vi "Fuzzy-Output-SubVi-2.0.vi"(0 "Slide in":refnum<vi>, 1 "Slide Refnum 4":refnum<vi>, 2 "Zero Upper Limit":dbl, 3 "Slide Refnum 5":refnum<vi>, 4 "Zero Medium Limit [Fixed]":dbl, 5 "Slide Refnum 6":refnum<vi>, 6 "Slide Refnum 7":refnum<vi>, 8 "Positive Lower Limit [Fixed]":dbl, 9 "Min Err":dbl, 10 "Slide Refnum 3":refnum<vi>, 11 "Negative Lower Limit [Fixed]":dbl, 12 "Positive Upper Limit [Fixed]":dbl, 13 "Negative Upper Limit [Fixed]":dbl, 14 "Slide Refnum in":refnum<vi>, 15 "Zero Lower Limit":dbl, 16 "Max Err":dbl, 18 "Min Intersection":dbl) -> (20 "Array":cluster{dbl[], dbl[]}[](array[cluster]))   [LabVIEW 2016]
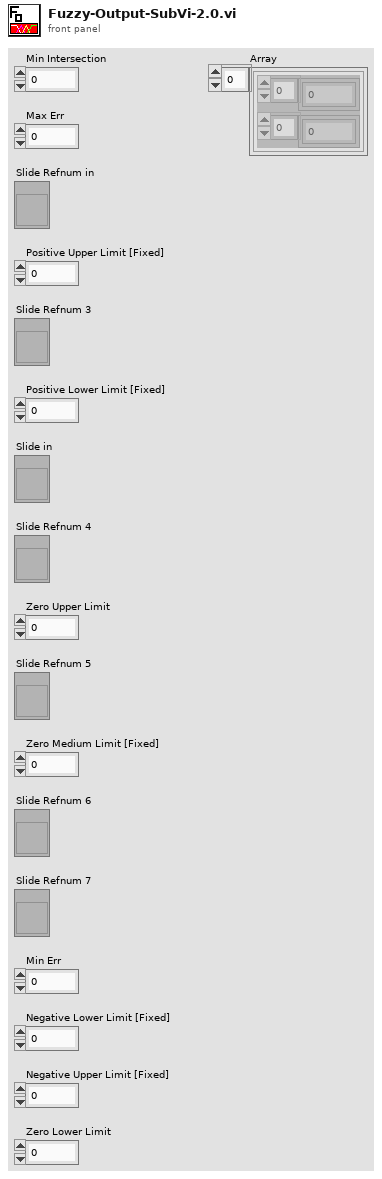
[diagram p1: front panel]
types:
  T1 = enum8{"Enabled", "Disabled", "Disabled and Grayed Out"}
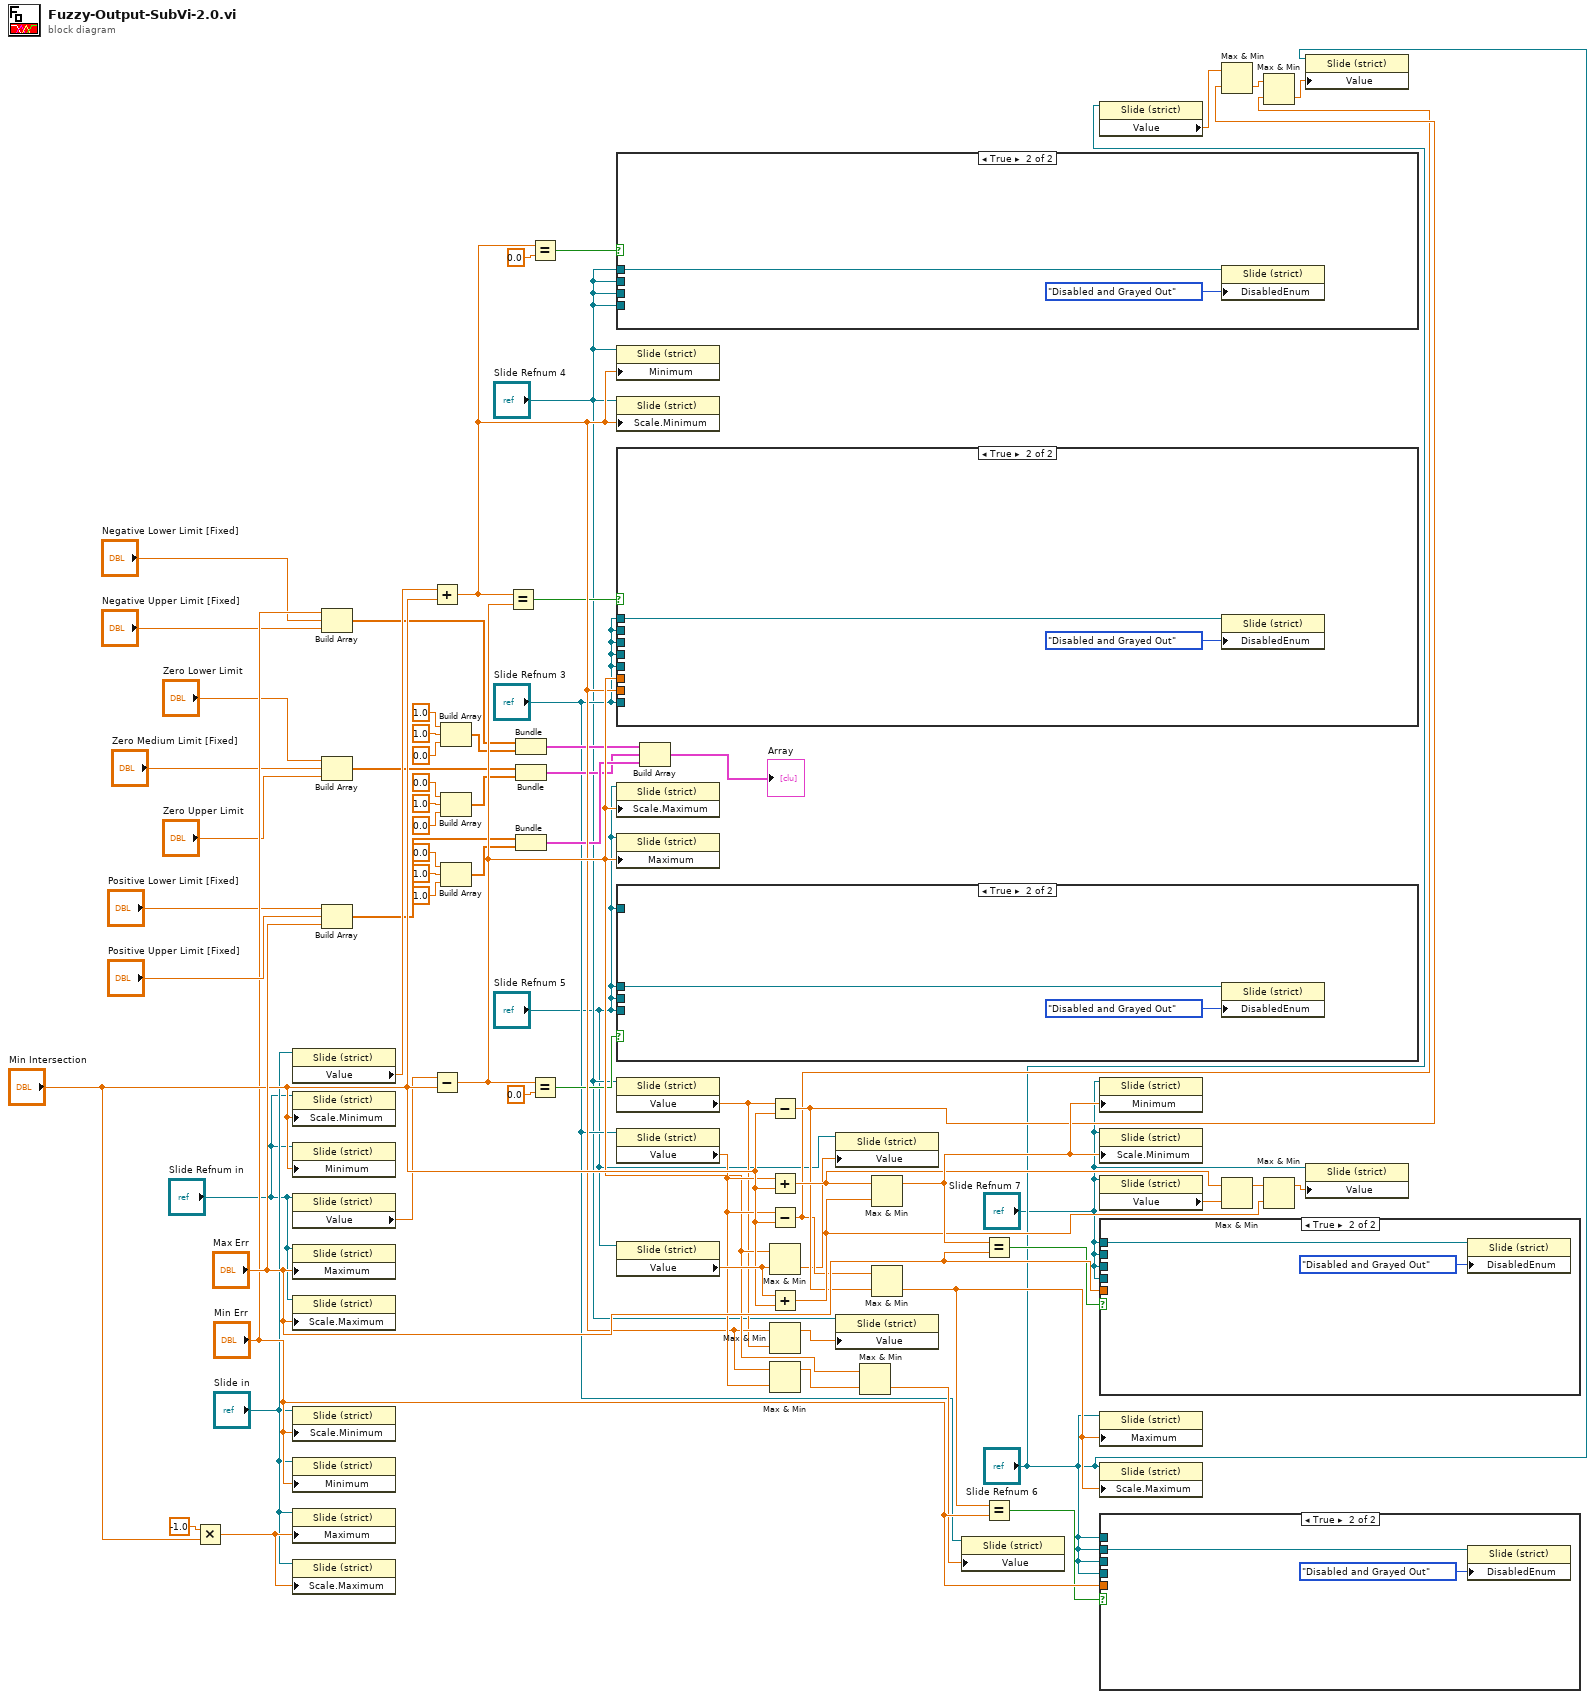
[diagram p0: block diagram]
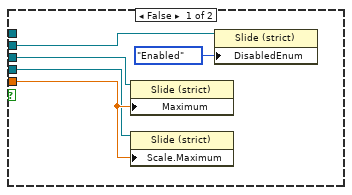
[diagram p2: hidden frame]
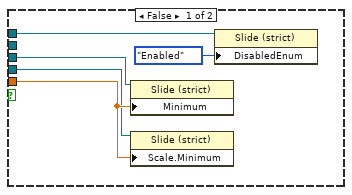
[diagram p3: hidden frame]
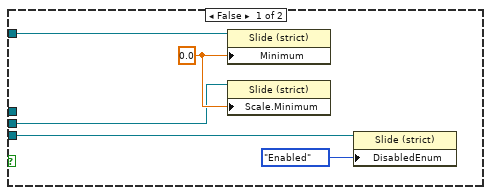
[diagram p4: hidden frame]
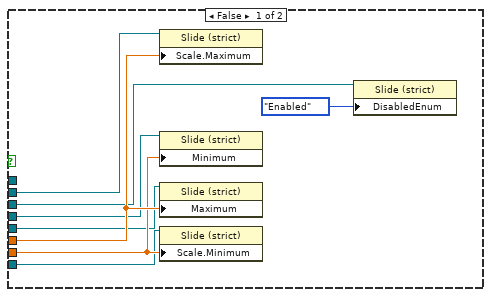
[diagram p5: hidden frame]
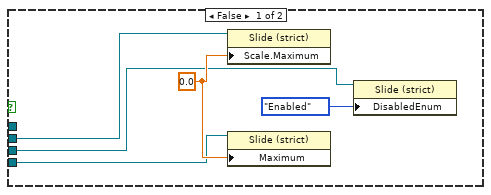
[diagram p6: hidden frame]
diagram:
  n1 = Multiply(x=-1.0, y="Min Intersection") -> (x*y=w54:dbl)
  n2 = property on="Property Node" class="Slide (strict)"(reference="Slide in") -> ("Value"=w32:dbl)  [unwired: 1 in, 2 out]
  n3 = property on="Property Node" class="Slide (strict)"(reference="Slide Refnum in", "Scale.Minimum"="Min Intersection") -> ()  [unwired: 1 in, 2 out]
  n4 = property on="Property Node" class="Slide (strict)"(reference="Slide Refnum in", "Minimum"="Min Intersection") -> ()  [unwired: 1 in, 2 out]
  n5 = property on="Property Node" class="Slide (strict)"(reference="Slide Refnum in") -> ("Value"=w31:dbl)  [unwired: 1 in, 2 out]
  n6 = property on="Property Node" class="Slide (strict)"(reference="Slide Refnum in", "Maximum"="Max Err") -> ()  [unwired: 1 in, 2 out]
  n7 = property on="Property Node" class="Slide (strict)"(reference="Slide Refnum in", "Scale.Maximum"="Max Err") -> ()  [unwired: 1 in, 2 out]
  n8 = property on="Property Node" class="Slide (strict)"(reference="Slide in", "Scale.Minimum"="Min Err") -> ()  [unwired: 1 in, 2 out]
  n9 = property on="Property Node" class="Slide (strict)"(reference="Slide in", "Minimum"="Min Err") -> ()  [unwired: 1 in, 2 out]
  n10 = property on="Property Node" class="Slide (strict)"(reference="Slide in", "Maximum"=w54) -> ()  [unwired: 1 in, 2 out]
  n11 = property on="Property Node" class="Slide (strict)"(reference="Slide in", "Scale.Maximum"=w54) -> ()  [unwired: 1 in, 2 out]
  n12 = Build Array("Min Err", "Negative Lower Limit [Fixed]", "Negative Upper Limit [Fixed]") -> (w10:dbl[])
  n13 = Build Array("Zero Lower Limit", "Zero Medium Limit [Fixed]", "Zero Upper Limit") -> (w18:dbl[])
  n14 = Build Array("Positive Lower Limit [Fixed]", "Positive Upper Limit [Fixed]", "Max Err") -> (w25:dbl[])
  n15 = Add(x=w32, y="Min Intersection") -> (x+y=w52:dbl)
  n16 = Subtract(x=w31, y="Min Intersection") -> (x-y=w55:dbl)
  n17 = Build Array(1.0 ("element"), 1.0 ("element"), 0.0 ("element")) -> (w11:dbl[])
  n18 = Build Array(0.0 ("element"), 1.0 ("element"), 0.0 ("element")) -> (w19:dbl[])
  n19 = Build Array(0.0 ("element"), 1.0 ("element"), 1.0 ("element")) -> (w26:dbl[])
  n20 = Equal?(x=w52, y=w55) -> (x = y?=w36:bool)
  n21 = Bundle(w10, w11) -> (w20:cluster{dbl[], dbl[]})  [unwired: 1 in]
  n22 = Bundle(w18, w19) -> (w21:cluster{dbl[], dbl[]})  [unwired: 1 in]
  n23 = Bundle(w25, w26) -> (w28:cluster{dbl[], dbl[]})  [unwired: 1 in]
  n24 = Equal?(x=w52, y=0.0) -> (x = y?=w35:bool)
  n25 = Equal?(x=w55, y=0.0) -> (x = y?=w39:bool)
  n26 = case shown="True" w35 {
    tunnel: "Slide Refnum 4" -> [w71 _]
    tunnel: "Slide Refnum 4" -> [w70 _]
    tunnel: "Slide Refnum 4" -> [w69 _]
    tunnel: "Slide Refnum 4" -> [_ w74]
    frame False {
      w72 = 0.0 ("Scale.Range:Maximum")
      n27 = property on="Property Node" class="Slide (strict)"(reference=w71, "Scale.Maximum"=w72) -> ()  [unwired: 1 in, 2 out]
      n28 = property on="Property Node" class="Slide (strict)"(reference=w69, "Maximum"=w72) -> ()  [unwired: 1 in, 2 out]
      n29 = property on="Property Node" class="Slide (strict)"(reference=w70, "DisabledEnum"=T1."Enabled" ("Disabled")) -> ()  [unwired: 1 in, 2 out]
    }
    frame True {
      n30 = property on="Property Node" class="Slide (strict)"(reference=w74, "DisabledEnum"=T1."Disabled and Grayed Out" ("Disabled")) -> ()  [unwired: 1 in, 2 out]
    }
  }
  n31 = property on="Property Node" class="Slide (strict)"(reference="Slide Refnum 4", "Minimum"=w52) -> ()  [unwired: 1 in, 2 out]
  n32 = property on="Property Node" class="Slide (strict)"(reference="Slide Refnum 4", "Scale.Minimum"=w52) -> ()  [unwired: 1 in, 2 out]
  n33 = case shown="True" w36 {
    tunnel: w52 -> [w81 _]
    tunnel: w55 -> [w82 _]
    tunnel: "Slide Refnum 3" -> [w80 _]
    tunnel: "Slide Refnum 3" -> [w79 _]
    tunnel: "Slide Refnum 3" -> [w78 _]
    tunnel: "Slide Refnum 3" -> [w77 _]
    tunnel: "Slide Refnum 3" -> [w76 _]
    tunnel: "Slide Refnum 3" -> [_ w84]
    frame False {
      n34 = property on="Property Node" class="Slide (strict)"(reference=w78, "Scale.Maximum"=w82) -> ()  [unwired: 1 in, 2 out]
      n35 = property on="Property Node" class="Slide (strict)"(reference=w76, "Minimum"=w81) -> ()  [unwired: 1 in, 2 out]
      n36 = property on="Property Node" class="Slide (strict)"(reference=w77, "Maximum"=w82) -> ()  [unwired: 1 in, 2 out]
      n37 = property on="Property Node" class="Slide (strict)"(reference=w79, "Scale.Minimum"=w81) -> ()  [unwired: 1 in, 2 out]
      n38 = property on="Property Node" class="Slide (strict)"(reference=w80, "DisabledEnum"=T1."Enabled" ("Disabled")) -> ()  [unwired: 1 in, 2 out]
    }
    frame True {
      n39 = property on="Property Node" class="Slide (strict)"(reference=w84, "DisabledEnum"=T1."Disabled and Grayed Out" ("Disabled")) -> ()  [unwired: 1 in, 2 out]
    }
  }
  n40 = property on="Property Node" class="Slide (strict)"(reference="Slide Refnum 5", "Scale.Maximum"=w55) -> ()  [unwired: 1 in, 2 out]
  n41 = property on="Property Node" class="Slide (strict)"(reference="Slide Refnum 5", "Maximum"=w55) -> ()  [unwired: 1 in, 2 out]
  n42 = case shown="True" w39 {
    tunnel: "Slide Refnum 5" -> [w88 _]
    tunnel: "Slide Refnum 5" -> [w87 _]
    tunnel: "Slide Refnum 5" -> [w86 _]
    tunnel: "Slide Refnum 5" -> [_ w91]
    frame False {
      w89 = 0.0 ("Scale.Range:Minimum")
      n43 = property on="Property Node" class="Slide (strict)"(reference=w86, "Minimum"=w89) -> ()  [unwired: 1 in, 2 out]
      n44 = property on="Property Node" class="Slide (strict)"(reference=w87, "Scale.Minimum"=w89) -> ()  [unwired: 1 in, 2 out]
      n45 = property on="Property Node" class="Slide (strict)"(reference=w88, "DisabledEnum"=T1."Enabled" ("Disabled")) -> ()  [unwired: 1 in, 2 out]
    }
    frame True {
      n46 = property on="Property Node" class="Slide (strict)"(reference=w91, "DisabledEnum"=T1."Disabled and Grayed Out" ("Disabled")) -> ()  [unwired: 1 in, 2 out]
    }
  }
  n47 = property on="Property Node" class="Slide (strict)"(reference="Slide Refnum 4") -> ("Value"=w45:dbl)  [unwired: 1 in, 2 out]
  n48 = property on="Property Node" class="Slide (strict)"(reference="Slide Refnum 3") -> ("Value"=w58:dbl)  [unwired: 1 in, 2 out]
  n49 = property on="Property Node" class="Slide (strict)"(reference="Slide Refnum 5") -> ("Value"=w62:dbl)  [unwired: 1 in, 2 out]
  n50 = Build Array(w20, w21, w28) -> (→"Array":cluster{dbl[], dbl[]}[])
  n51 = Subtract(x=w45, y="Min Intersection") -> (x-y=w49:dbl)
  n52 = Add(x=w58, y="Min Intersection") -> (x+y=w64:dbl)
  n53 = Subtract(x=w58, y="Min Intersection") -> (x-y=w48:dbl)
  n54 = Max & Min(x=w55, y=w62) -> (min(x,y)=w37:dbl)  [unwired: 1 out]
  n55 = Add(x=w62, y="Min Intersection") -> (x+y=w65:dbl)
  n56 = Max & Min(x=w52, y=w45) -> (max(x,y)=w33:dbl)  [unwired: 1 out]
  n57 = Max & Min(x=w52, y=w58) -> (max(x,y)=w30:dbl)  [unwired: 1 out]
  n58 = property on="Property Node" class="Slide (strict)"(reference="Slide Refnum 5", "Value"=w37) -> ()  [unwired: 1 in, 2 out]
  n59 = property on="Property Node" class="Slide (strict)"(reference="Slide Refnum 4", "Value"=w33) -> ()  [unwired: 1 in, 2 out]
  n60 = Max & Min(x=w55, y=w30) -> (min(x,y)=w29:dbl)  [unwired: 1 out]
  n61 = Max & Min(x=w64, y=w65) -> (max(x,y)=w66:dbl)  [unwired: 1 out]
  n62 = Max & Min(x=w48, y=w49) -> (min(x,y)=w51:dbl)  [unwired: 1 out]
  n63 = property on="Property Node" class="Slide (strict)"(reference="Slide Refnum 3", "Value"=w29) -> ()  [unwired: 1 in, 2 out]
  n64 = Equal?(x=w66, y="Max Err") -> (x = y?=w67:bool)
  n65 = Equal?(x=w51, y="Min Err") -> (x = y?=w50:bool)
  n66 = property on="Property Node" class="Slide (strict)"(reference="Slide Refnum 6") -> ("Value"=w44:dbl)  [unwired: 1 in, 2 out]
  n67 = property on="Property Node" class="Slide (strict)"(reference="Slide Refnum 7", "Minimum"=w66) -> ()  [unwired: 1 in, 2 out]
  n68 = property on="Property Node" class="Slide (strict)"(reference="Slide Refnum 7", "Scale.Minimum"=w66) -> ()  [unwired: 1 in, 2 out]
  n69 = property on="Property Node" class="Slide (strict)"(reference="Slide Refnum 7") -> ("Value"=w59:dbl)  [unwired: 1 in, 2 out]
  n70 = case shown="True" w67 {
    tunnel: "Max Err" -> [w96 _]
    tunnel: "Slide Refnum 7" -> [w95 _]
    tunnel: "Slide Refnum 7" -> [w94 _]
    tunnel: "Slide Refnum 7" -> [w93 _]
    tunnel: "Slide Refnum 7" -> [_ w98]
    frame False {
      n71 = property on="Property Node" class="Slide (strict)"(reference=w94, "Maximum"=w96) -> ()  [unwired: 1 in, 2 out]
      n72 = property on="Property Node" class="Slide (strict)"(reference=w93, "Scale.Maximum"=w96) -> ()  [unwired: 1 in, 2 out]
      n73 = property on="Property Node" class="Slide (strict)"(reference=w95, "DisabledEnum"=T1."Enabled" ("Disabled")) -> ()  [unwired: 1 in, 2 out]
    }
    frame True {
      n74 = property on="Property Node" class="Slide (strict)"(reference=w98, "DisabledEnum"=T1."Disabled and Grayed Out" ("Disabled")) -> ()  [unwired: 1 in, 2 out]
    }
  }
  n75 = property on="Property Node" class="Slide (strict)"(reference="Slide Refnum 6", "Maximum"=w51) -> ()  [unwired: 1 in, 2 out]
  n76 = property on="Property Node" class="Slide (strict)"(reference="Slide Refnum 6", "Scale.Maximum"=w51) -> ()  [unwired: 1 in, 2 out]
  n77 = case shown="True" w50 {
    tunnel: "Min Err" -> [w103 _]
    tunnel: "Slide Refnum 6" -> [w102 _]
    tunnel: "Slide Refnum 6" -> [w101 _]
    tunnel: "Slide Refnum 6" -> [w100 _]
    tunnel: "Slide Refnum 6" -> [_ w105]
    frame False {
      n78 = property on="Property Node" class="Slide (strict)"(reference=w100, "Minimum"=w103) -> ()  [unwired: 1 in, 2 out]
      n79 = property on="Property Node" class="Slide (strict)"(reference=w101, "Scale.Minimum"=w103) -> ()  [unwired: 1 in, 2 out]
      n80 = property on="Property Node" class="Slide (strict)"(reference=w102, "DisabledEnum"=T1."Enabled" ("Disabled")) -> ()  [unwired: 1 in, 2 out]
    }
    frame True {
      n81 = property on="Property Node" class="Slide (strict)"(reference=w105, "DisabledEnum"=T1."Disabled and Grayed Out" ("Disabled")) -> ()  [unwired: 1 in, 2 out]
    }
  }
  n82 = Max & Min(x=w44, y=w49) -> (min(x,y)=w46:dbl)  [unwired: 1 out]
  n83 = Max & Min(x=w64, y=w59) -> (max(x,y)=w61:dbl)  [unwired: 1 out]
  n84 = Max & Min(x=w46, y=w48) -> (min(x,y)=w47:dbl)  [unwired: 1 out]
  n85 = Max & Min(x=w61, y=w65) -> (max(x,y)=w63:dbl)  [unwired: 1 out]
  n86 = property on="Property Node" class="Slide (strict)"(reference="Slide Refnum 6", "Value"=w47) -> ()  [unwired: 1 in, 2 out]
  n87 = property on="Property Node" class="Slide (strict)"(reference="Slide Refnum 7", "Value"=w63) -> ()  [unwired: 1 in, 2 out]
